vi "InitADCHannel.vi"(1 "error out":errorcluster) -> (0 "Boolean":bool, 2 "number":i32, 3 "DLL error code":u32, 4 "String":string, 5 "error out 2":errorcluster)   [LabVIEW 2011]
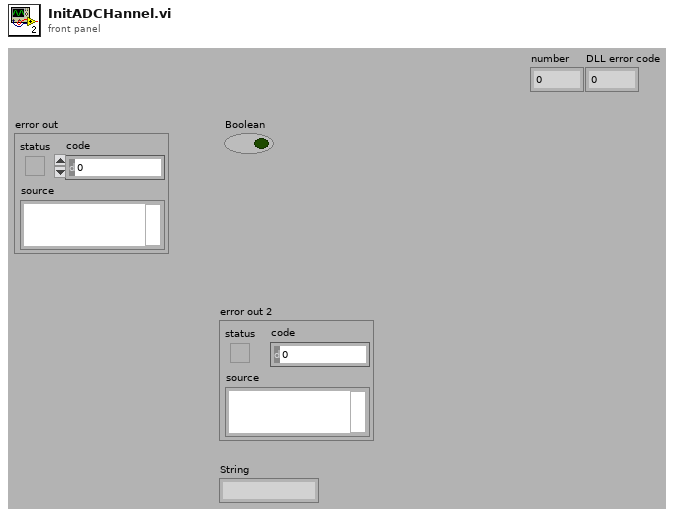
[diagram p1: front panel]
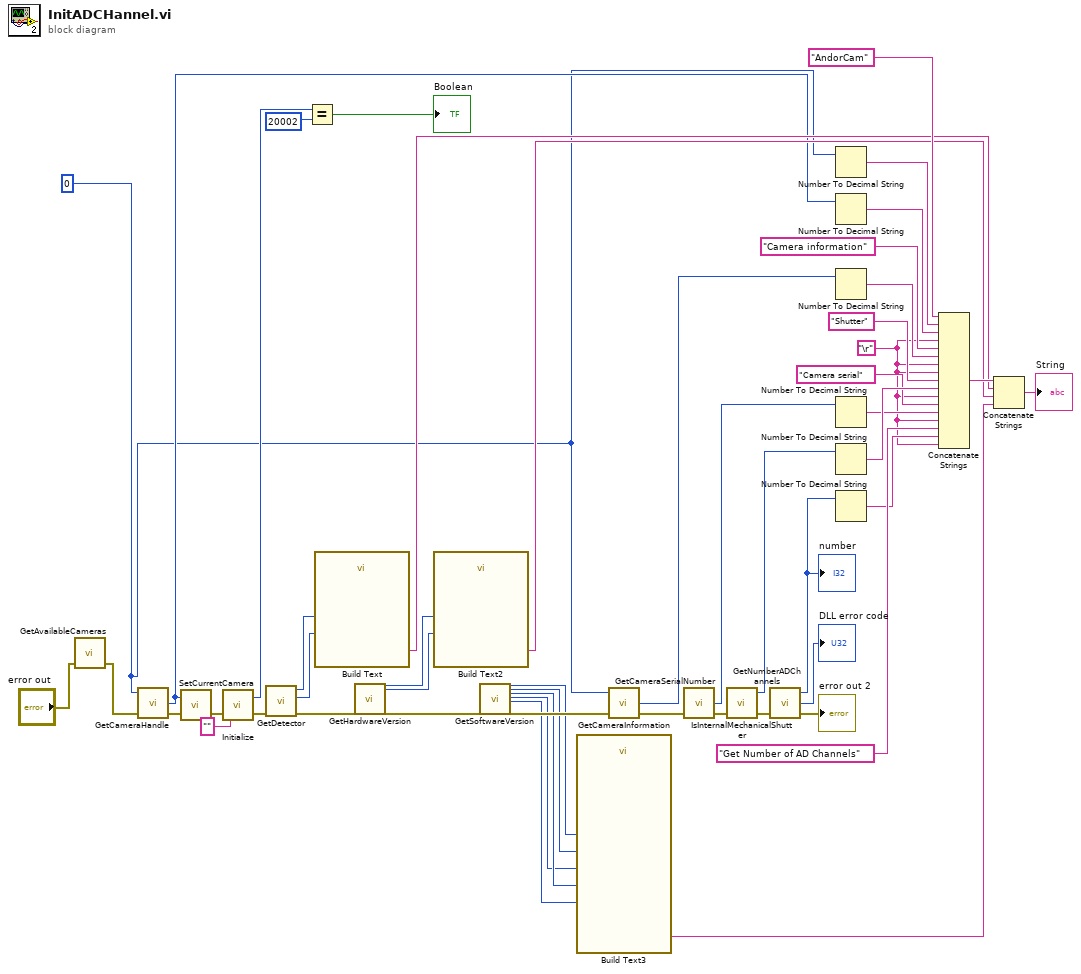
[diagram p0: block diagram]
diagram:
  w2 = 0
  w14 = "\r"
  n1 = call "GetAvailableCameras.vi"("error in (no error)"="error out") -> ("error out"=w4:errorcluster)  [unwired: 2 in, 2 out]
  n2 = call "GetCameraHandle.vi"("error in (no error)"=w4, "cameraIndex"=w2) -> ("error out"=w43:errorcluster, "cameraHandle"=w3:i32)  [unwired: 1 in, 1 out]
  n3 = call "SetCurrentCamera.vi"("error in (no error)"=w43, "cameraHandle"=w3) -> ("error out"=w42:errorcluster)  [unwired: 1 out]
  n4 = call "Initialize.vi"("error in (no error)"=w42, "directory (\"\")"="" ("directory (\"\")")) -> ("error out"=w44:errorcluster, "DLL error code"=w13:u32)
  n5 = call "GetDetector.vi"("error in (no error)"=w44) -> ("error out"=w45:errorcluster, "ypixels"=w34:i32, "xpixels"=w35:i32)  [unwired: 3 in, 1 out]
  n6 = Equal?(x=w13, y=u32 20002) -> (x = y?=→"Boolean":bool)
  n7 = call "Build Text"("x"=w35, "y"=w34) -> ("Result"=w11:string)  [unwired: 12 in, 1 out]
  n8 = call "GetHardwareVersion.vi"("error in (no error)"=w45) -> ("PCB"=w33:u32, "Flex"=w32:u32, "error out"=w41:errorcluster)  [unwired: 19 in, 5 out]
  n9 = call "Build Text2"("pcb"=w33, "FLEX"=w32) -> ("Result"=w10:string)  [unwired: 12 in, 1 out]
  n10 = call "GetSoftwareVersion.vi"("error in (no error)"=w41) -> ("eprom"=w31:u32, "cofFile"=w30:u32, "vxdRev"=w29:u32, "vxdVer"=w28:u32, "dllRev"=w27:u32, "error out"=w46:errorcluster)  [unwired: 19 in, 2 out]
  n11 = call "Build Text3"("vxdrew"=w29, "eprom"=w31, "con"=w30, "vxdver"=w28, "dllrev"=w27) -> ("Result"=w9:string)  [unwired: 9 in, 1 out]
  n12 = call "GetCameraInformation.vi"("error in (no error)"=w46, "index"=w2) -> ("error out"=w40:errorcluster, "information"=w24:i32)  [unwired: 1 in, 1 out]
  n13 = call "GetCameraSerialNumber.vi"("error in (no error)"=w40) -> ("error out"=w6:errorcluster, "number"=w18:i32)  [unwired: 2 in, 1 out]
  n14 = call "IsInternalMechanicalShutter.vi"("error in (no error)"=w6) -> ("error out"=w49:errorcluster, "DLL error code"=w21:u32)  [unwired: 2 in, 1 out]
  n15 = call "GetNumberADChannels.vi"("error in (no error)"=w49) -> ("error out"=→"error out 2":errorcluster, "DLL error code"=→"DLL error code":u32, "number"=w16:i32)  [unwired: 2 in]
  "number" <- w16
  n16 = Number To Decimal String(number=w2) -> (decimal integer string=w48:string)  [unwired: 1 in]
  n17 = Number To Decimal String(number=w3) -> (decimal integer string=w36:string)  [unwired: 1 in]
  n18 = Number To Decimal String(number=w24) -> (decimal integer string=w25:string)  [unwired: 1 in]
  n19 = Number To Decimal String(number=w18) -> (decimal integer string=w19:string)  [unwired: 1 in]
  n20 = Number To Decimal String(number=w21) -> (decimal integer string=w22:string)  [unwired: 1 in]
  n21 = Number To Decimal String(number=w16) -> (decimal integer string=w15:string)  [unwired: 1 in]
  n22 = Concatenate Strings("AndorCam" ("directory (\"\")"), w48, w36, w14, "Camera information" ("string"), w25, w14, w14, "Shutter" ("string"), w22, w14, "Camera serial" ("string"), w19, w14, "Get Number of AD Channels" ("string"), w15, w14) -> (w12:string)
  n23 = Concatenate Strings(w12, w11, w10, w9) -> (→"String":string)
